vi "SaveDialog.vi"(8 "error in":errorcluster, 10 "current path":path, 11 "repository":refnum<class "CEF_Repository.lvclass">) -> (0 "error out":errorcluster, 2 "Done?":bool, 3 "repository out":refnum<class "CEF_Repository.lvclass">)   [LabVIEW 2025, in "Config Tool.lvlib"]
doc: "This VI ask if you want to save the changes. Depending on the response and the validity of the ccurrent path, it will save the configuration or display the save as dialog.Copyright 2017 National Instruments Corporation\n\nLicensed under the Apache License, Version 2.0 (the \"License\"); you may not use this file except in compliance with the License. You may obtain a copy of the License at http://www.apache.org/licenses/LICENSE-2.0\nUnless required by applicable law or agreed to in writing, software distributed under the License is distributed on an \"AS IS\" BASIS, WITHOUT WARRANTIES OR CONDITIONS OF ANY KIND, either express or implied. See the License for the specific language governing permissions and limitations under the License."
uses:
  Config Tool.lvlib
  Users/Public/Documents/Sandia National Labs/TSS Plugin/CEF.lvlibp/Repository/CEF_Repository.lvclass
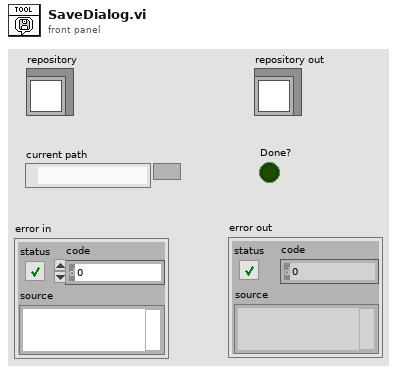
[diagram p1: front panel]
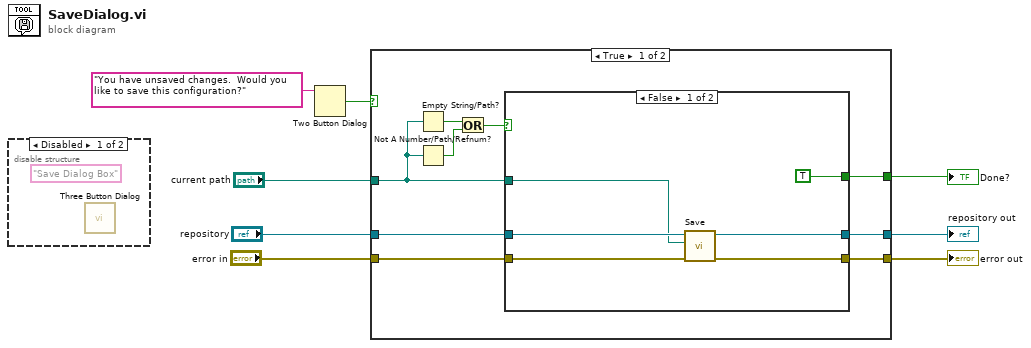
[diagram p0: block diagram]
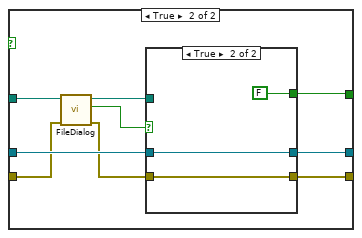
[diagram p3: hidden frame]
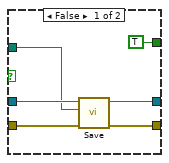
[diagram p4: hidden frame]
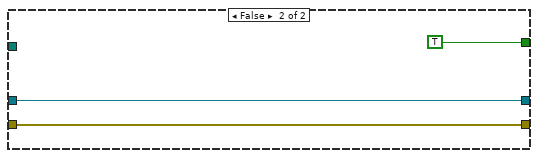
[diagram p5: hidden frame]
diagram:
  n1 = disable-structure shown="Disabled" {
    frame Disabled {
      (unwired) "Save Dialog Box" ("Window Title (\"\")")
      n2 = call <vilib>:"Three Button Dialog.vi"() -> ()  [unwired: 11 in, 1 out]
    }
    frame Enabled {
    }
  }
  n3 = Two Button Dialog(message="You have unsaved changes.  Would you like to save this configuration?") -> (T button?=w1:bool)  [unwired: 2 in]
  n4 = case shown="True" w1 {
    tunnel: [w10 w42] -> w5
    tunnel: "error in" -> [w14 w43]
    tunnel: [w13 w43] -> w7
    tunnel: [w9 TRUE ("New")] -> w6
    tunnel: "repository" -> [w11 w42]
    tunnel: "current path" -> [w12 _]
    frame True {
      n5 = Empty String/Path?(string/path=w12) -> (empty?=w16:bool)
      n6 = Not A Number/Path/Refnum?(number/path/refnum=w12) -> (NaN/Path/Refnum?=w17:bool)
      n7 = Or(x=w16, y=w17) -> (x .or. y?=w15:bool)
      n8 = case shown="False" w15 {
        tunnel: w12 -> [w21 w25]
        tunnel: w14 -> [w23 w27]
        tunnel: w11 -> [w22 w30]
        tunnel: [w19 w29] -> w10
        tunnel: [w20 w28] -> w13
        tunnel: [TRUE ("New") w24] -> w9
        frame False {
          # "unchanged file path"
          n9 = call-dynamic "Save.vi"("error in"=w23, "file path"=w21, "CEF_Repository in"=w22) -> ("error out"=w20:errorcluster, "CEF_Repository out"=w19:refnum<class "CEF_Repository.lvclass">)  [unwired: 7 in]
        }
        frame True {
          # "Empthy path, Not a Path, and changed"
          n10 = call "FileDialog.vi"("error in"=w27, "start path"=w25) -> ("error out"=w26:errorcluster, "cancelled"=w32:bool, "selected path"=w31:path)  [unwired: 7 in]
          n11 = case shown="True" w32 {
            tunnel: w31 -> [w36 _]
            tunnel: w26 -> [w38 w40]
            tunnel: w30 -> [w37 w41]
            tunnel: [w35 w41] -> w29
            tunnel: [w34 w40] -> w28
            tunnel: [TRUE ("New") FALSE ("New")] -> w24
            frame False {
              n12 = call-dynamic "Save.vi"("error in"=w38, "file path"=w36, "CEF_Repository in"=w37) -> ("error out"=w34:errorcluster, "CEF_Repository out"=w35:refnum<class "CEF_Repository.lvclass">)  [unwired: 7 in]
            }
            frame True {
            }
          }
        }
      }
    }
    frame False {
    }
  }
  "error out" <- w7
  "Done?" <- w6
  "repository out" <- w5
